vi "Dilution_visible_01.vi"(1 "calculated":u16, 2 "dilution":bool) -> (0 "Visible":T1)   [LabVIEW 2011]
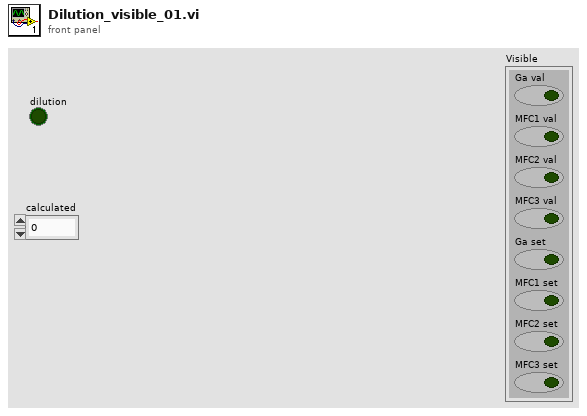
[diagram p1: front panel]
types:
  T1 = cluster{"Ga val":bool, "MFC1 val":bool, "MFC2 val":bool, "MFC3 val":bool, "Ga set":bool, "MFC1 set":bool, "MFC2 set":bool, "MFC3 set":bool}
  T2 = cluster{"Visible":bool, "Visible":bool, "Visible":bool, "Visible":bool, "Visible":bool, "Visible":bool, "Visible":bool, "Visible":bool}
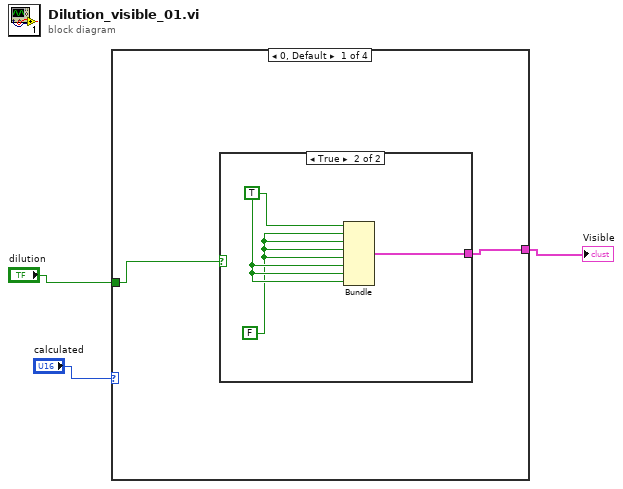
[diagram p0: block diagram]
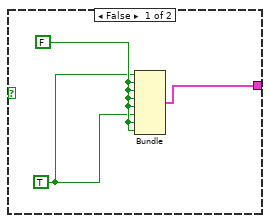
[diagram p2: hidden frame]
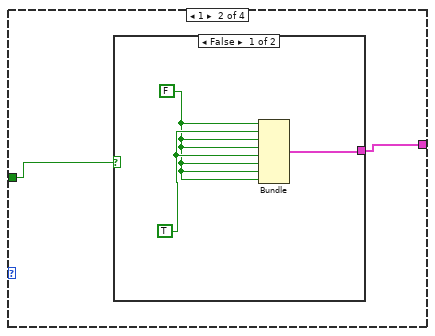
[diagram p3: hidden frame]
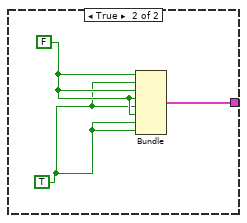
[diagram p4: hidden frame]
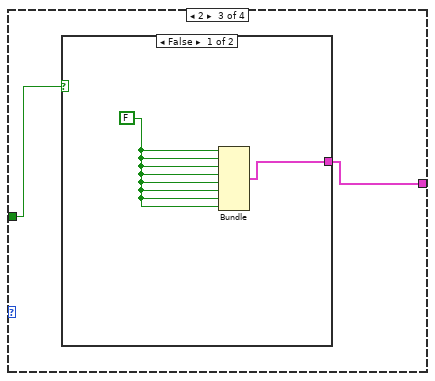
[diagram p5: hidden frame]
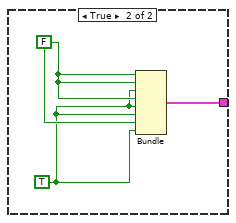
[diagram p6: hidden frame]
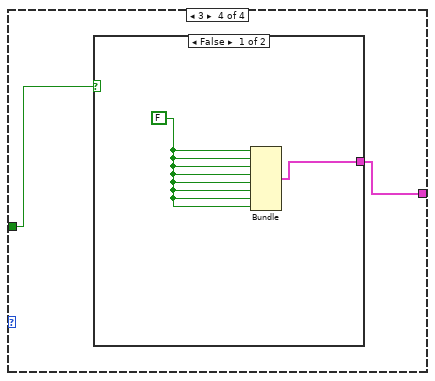
[diagram p7: hidden frame]
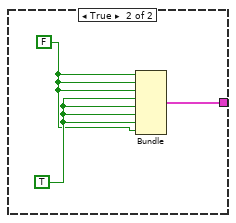
[diagram p8: hidden frame]
diagram:
  n1 = case shown="0, Default" "calculated" {
    tunnel: "dilution" -> [w4 w13 w20 w28]
    tunnel: [w5 w12 w21 w27] -> w1
    frame 0, Default {
      n2 = case shown="True" w4 {
        tunnel: [w8 w11] -> w5
        frame False {
          w6 = TRUE ("Visible")
          w7 = FALSE ("Visible")
          n3 = Bundle("Visible"=w6, "Visible"=w7, "Visible"=w7, "Visible"=w7, "Visible"=w7, "Visible"=w6, "Visible"=w7, "Visible"=w7) -> (w8:T2)  [unwired: 1 in]
        }
        frame True {
          w9 = FALSE ("Visible")
          w10 = TRUE ("Visible")
          n4 = Bundle("Visible"=w10, "Visible"=w9, "Visible"=w9, "Visible"=w9, "Visible"=w9, "Visible"=w10, "Visible"=w10, "Visible"=w10) -> (w11:T2)  [unwired: 1 in]
        }
      }
    }
    frame 1 {
      n5 = case shown="False" w13 {
        tunnel: [w16 w19] -> w12
        frame False {
          w15 = TRUE ("Visible")
          w14 = FALSE ("Visible")
          n6 = Bundle("Visible"=w14, "Visible"=w15, "Visible"=w14, "Visible"=w14, "Visible"=w15, "Visible"=w14, "Visible"=w14, "Visible"=w14) -> (w16:T2)  [unwired: 1 in]
        }
        frame True {
          w17 = TRUE ("Visible")
          w18 = FALSE ("Visible")
          n7 = Bundle("Visible"=w18, "Visible"=w17, "Visible"=w18, "Visible"=w18, "Visible"=w17, "Visible"=w18, "Visible"=w17, "Visible"=w17) -> (w19:T2)  [unwired: 1 in]
        }
      }
    }
    frame 2 {
      n8 = case shown="False" w20 {
        tunnel: [w23 w26] -> w21
        frame False {
          w22 = FALSE ("Visible")
          n9 = Bundle("Visible"=w22, "Visible"=w22, "Visible"=w22, "Visible"=w22, "Visible"=w22, "Visible"=w22, "Visible"=w22, "Visible"=w22) -> (w23:T2)  [unwired: 1 in]
        }
        frame True {
          w24 = TRUE ("Visible")
          w25 = FALSE ("Visible")
          n10 = Bundle("Visible"=w25, "Visible"=w25, "Visible"=w24, "Visible"=w25, "Visible"=w24, "Visible"=w24, "Visible"=w25, "Visible"=w24) -> (w26:T2)  [unwired: 1 in]
        }
      }
    }
    frame 3 {
      n11 = case shown="False" w28 {
        tunnel: [w30 w33] -> w27
        frame False {
          w29 = FALSE ("Visible")
          n12 = Bundle("Visible"=w29, "Visible"=w29, "Visible"=w29, "Visible"=w29, "Visible"=w29, "Visible"=w29, "Visible"=w29, "Visible"=w29) -> (w30:T2)  [unwired: 1 in]
        }
        frame True {
          w32 = TRUE ("Visible")
          w31 = FALSE ("Visible")
          n13 = Bundle("Visible"=w31, "Visible"=w31, "Visible"=w31, "Visible"=w32, "Visible"=w32, "Visible"=w32, "Visible"=w32, "Visible"=w31) -> (w33:T2)  [unwired: 1 in]
        }
      }
    }
  }
  "Visible" <- w1
